vi "problem2.vi"() -> ()   [LabVIEW 2017]
panel:
  out "Numeric":dbl
  out "Boolean 5":bool
  in  "stop":bool
  in  "Boolean 4":bool
  in  "Boolean 3":bool
  in  "Boolean 2":bool
  in  "Boolean":bool
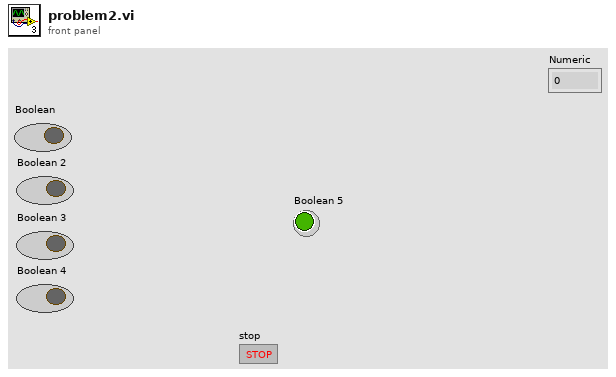
[diagram p1: front panel]
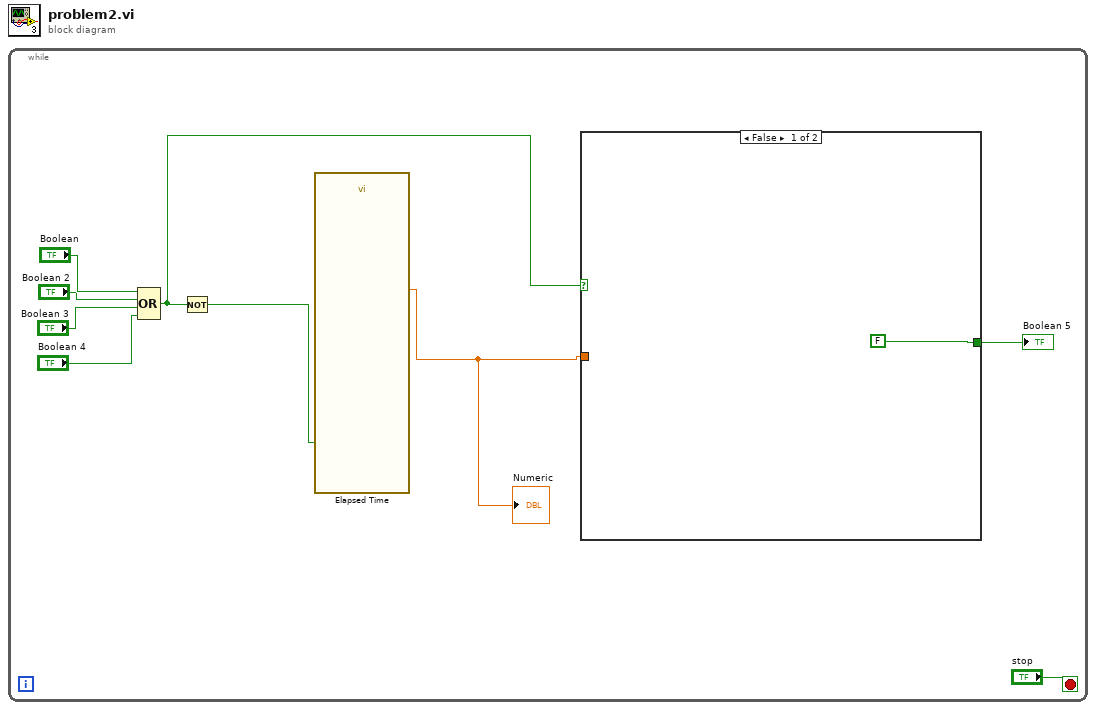
[diagram p0: block diagram]
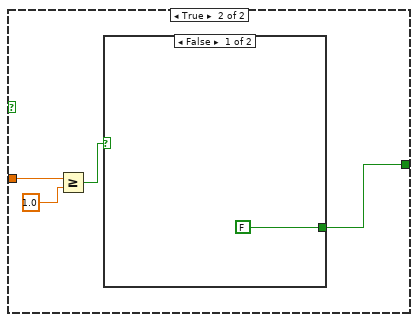
[diagram p2: hidden frame]
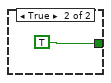
[diagram p3: hidden frame]
diagram:
  n1 = while {
    stop <- "stop" stop-if-true
    n2 = Compound Arithmetic op=OR("Boolean", "Boolean 2", "Boolean 3", "Boolean 4") -> (w3:bool)
    n3 = Not(x=w3) -> (.not. x?=w4:bool)
    n4 = call "Elapsed Time"("Reset"=w4) -> ("Elapsed Time (s)"=w1:dbl)  [unwired: 11 in, 7 out]
    "Numeric" <- w1
    n5 = case shown="False" w3 {
      tunnel: w1 -> [_ w11]
      tunnel: [FALSE w14] -> w2
      frame False {
      }
      frame True {
        n6 = Greater Or Equal?(x=w11, y=1.0 ("x")) -> (x >= y?=w13:bool)
        n7 = case shown="False" w13 {
          tunnel: [FALSE TRUE] -> w14
          frame False {
          }
          frame True {
          }
        }
      }
    }
    "Boolean 5" <- w2
  }
